vi "PRIME Telescope Configure GUI.vi"(11 "Settings":T1) -> (3 "Settings out":T1)   [LabVIEW 2021, in "PRIME Telescope.lvclass"]
uses:
  PRIME Telescope.lvclass
  PRIME Telescope cluster Settings.ctl
panel:
  in  "Cancel Button":bool
  in  "OK Button":bool
  in  "remote port":u16
  in  "IP Address":string
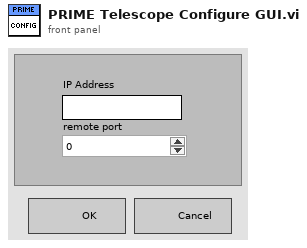
[diagram p1: front panel]
types:
  T1 = typedef "PRIME Telescope cluster Settings.ctl" = cluster{"IP Address":string, "port":u16}
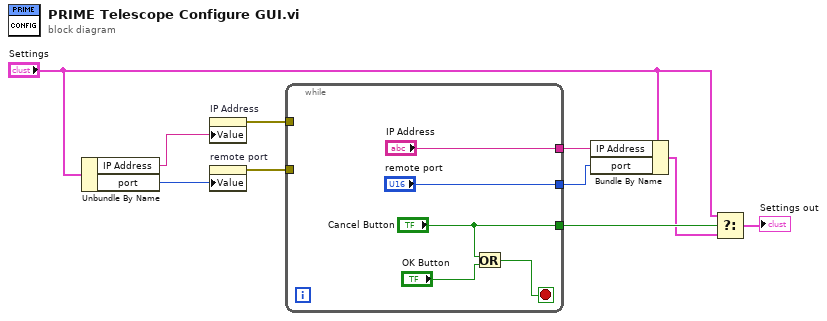
[diagram p0: block diagram]
diagram:
  n1 = Unbundle By Name("Settings") -> ("IP Address"=w10:string, "port"=w9:u16)
  n2 = property on="IP Address" class="Str"("Value"=w10) -> (error out=w8:errorcluster)  [unwired: 2 in, 1 out]
  n3 = property on="remote port" class="DigNum (strict)"("Value"=w9) -> (error out=w7:errorcluster)  [unwired: 2 in, 1 out]
  n4 = while {
    tunnel: ["Cancel Button"] -> w4
    tunnel: w8 -> [_]
    tunnel: w7 -> [_]
    tunnel: ["IP Address"] -> w6
    tunnel: ["remote port"] -> w5
    stop <- w14 stop-if-true
    n5 = Or(x="Cancel Button", y="OK Button") -> (x .or. y?=w14:bool)
  }
  n6 = Bundle By Name(cluster="Settings", "IP Address"=w6, "port"=w5) -> (w2:T1)
  n7 = Select(t="Settings", s=w4, f=w2) -> (s? t:f=→"Settings out":T1)
